vi "LibXML_IndexNodeList.vi"(8 "error in":errorcluster, 10 "index":i32, 11 "XPathObj":u32) -> (0 "error out":errorcluster, 2 "NodePtr":u32, 3 "XPathObj out":u32)   [LabVIEW 2019, in "Tools.lvlib" / "LibXML.lvlib"]
doc: "Gets a node pointer (U32) to the node at index"
uses:
  LibXML.lvlib
  <vilib>/Utility/error.llb/Trim Whitespace.vi
  Tools.lvlib
  dll/lXMLwrap.dll
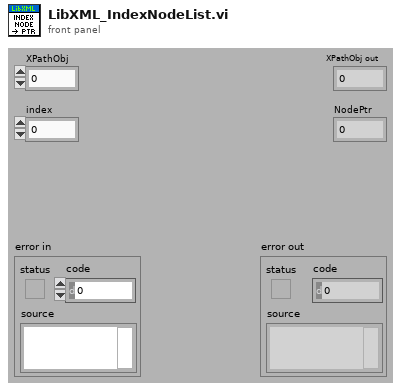
[diagram p1: front panel]
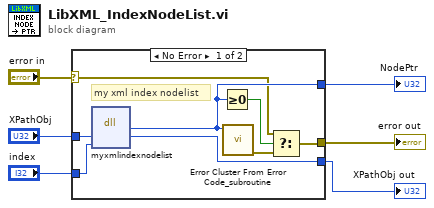
[diagram p0: block diagram]
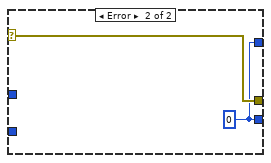
[diagram p2: hidden frame]
diagram:
  n1 = case shown="No Error" "error in" {
    selector: "error in" -> [w7 w16]
    tunnel: [w13 w16] -> w5
    tunnel: [w11 w15] -> w4
    tunnel: "XPathObj" -> [w10 _]
    tunnel: "index" -> [w9 _]
    tunnel: [w8 w15] -> w1
    frame No Error {
      # "my xml index nodelist"
      n2 = dll-call lib="C:/Projects/_Prywatne/MyCIT/Framework/Tools/XML/LibXML/dll/lXMLwrap.dll" fn="myxmlindexnodelist"("nodesetptr"=w10, "index"=w9) -> ("return type"=w11:u32, "nodesetptr"=w8:u32)  [unwired: 4 in, 2 out]
      n3 = Greater Or Equal To 0?(x=w11) -> (x >= 0?=w14:bool)
      n4 = call "Error Cluster From Error Code_subroutine.vi"("error code (0)"=w11) -> ("error out"=w12:errorcluster)  [unwired: 8 in]
      n5 = Select(t=w7, s=w14, f=w12) -> (s? t:f=w13:errorcluster)
    }
    frame Error {
      w15 = u32 0
    }
  }
  "error out" <- w5
  "NodePtr" <- w4
  "XPathObj out" <- w1
